vi "Trace.vi"(8 "Error In":errorcluster, 11 "Message":string) -> (0 "Error Out":errorcluster)   [LabVIEW 2014, in "LV-Logger.lvlib"]
uses:
  LV-Logger.lvlib
  Action.ctl
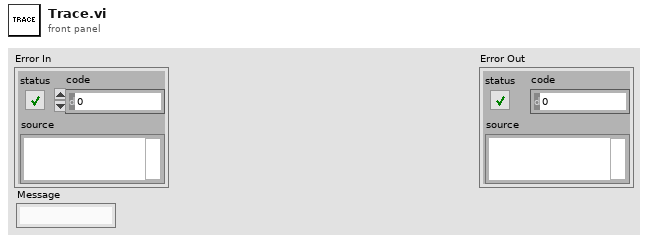
[diagram p1: front panel]
types:
  T1 = typedef "LV-Logger.lvlib/Action.ctl" = enum16{"Initialize", "Get", "Fatal", "Error", "Debug", "Warn", "Info", "Trace", "Shutdown"}
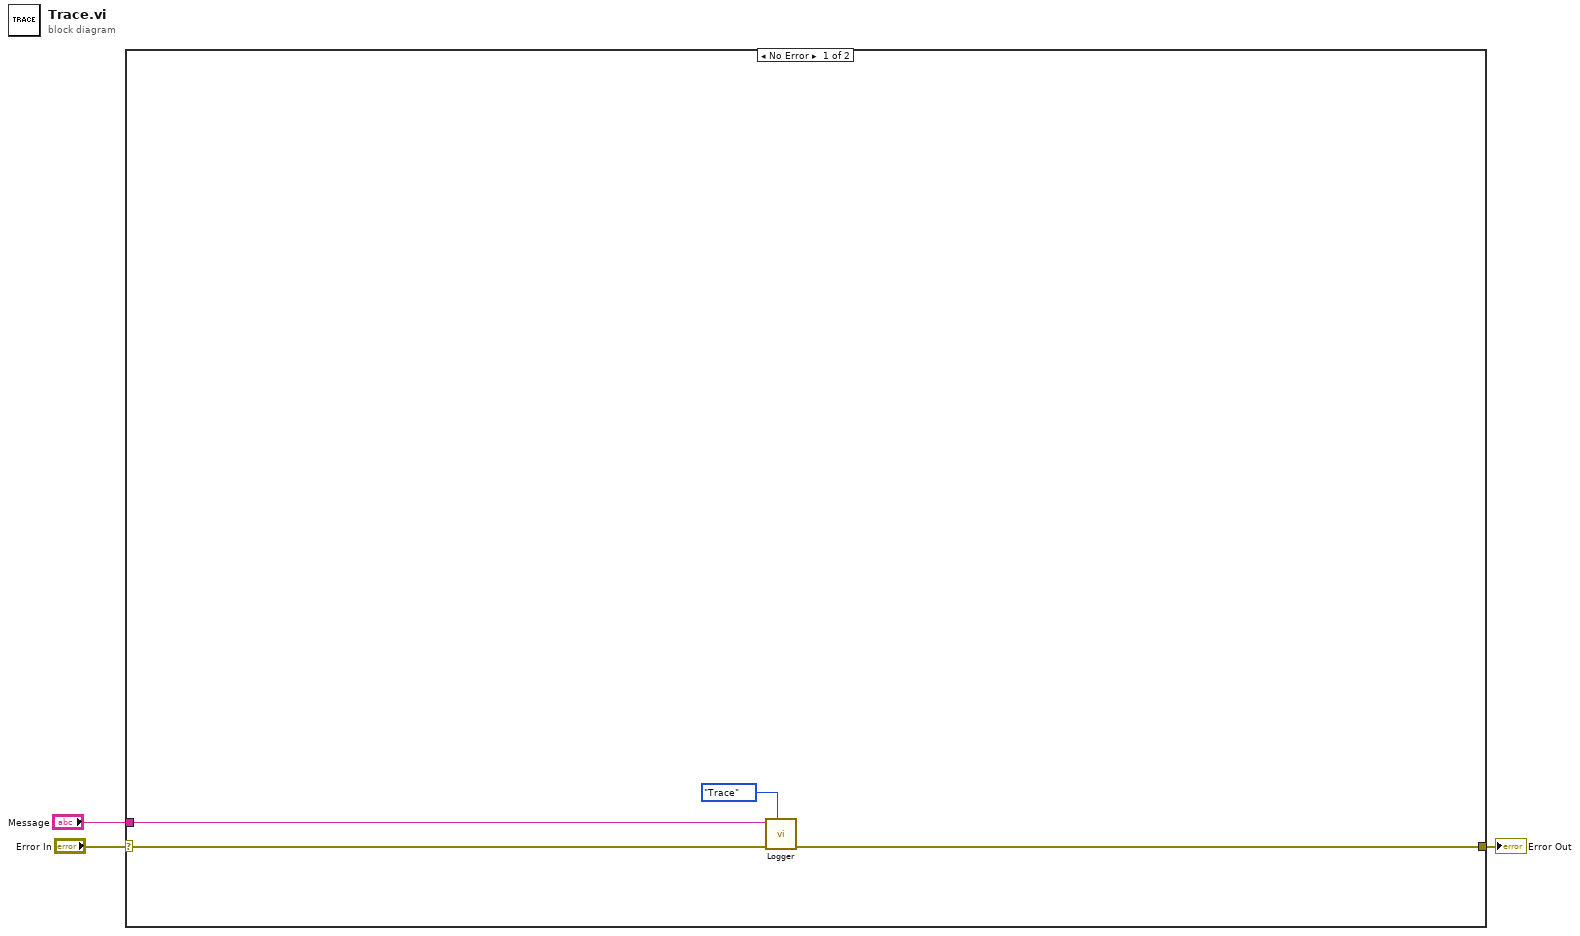
[diagram p0: block diagram]
diagram:
  n1 = case shown="No Error" "Error In" {
    selector: "Error In" -> [w7 w8]
    tunnel: [w6 w8] -> w2
    tunnel: "Message" -> [w5 _]
    frame No Error {
      n2 = call "Logger.vi"("Action"=Action."Trace", "Error In"=w7, "Message"=w5) -> ("Error Out"=w6:errorcluster)  [unwired: 7 in, 1 out]
    }
    frame Error {
    }
  }
  "Error Out" <- w2
